vi "tmx-in-range.vi"(3 "high":u16=160, 4 "input":u16=160, 5 "low":u16=60) -> (1 "result":bool)   [LabVIEW 2010]
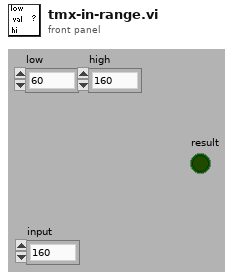
[diagram p1: front panel]
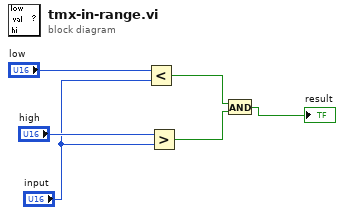
[diagram p0: block diagram]
diagram:
  n1 = Less?(x="low", y="input") -> (x < y?=w3:bool)
  n2 = Greater?(x="high", y="input") -> (0:w2:bool)
  n3 = And(x=w3, y=w2) -> (x .and. y?=→"result":bool)
